vi "Global 6 Bool.vi"() -> ()   [LabVIEW 2022 SP3]
panel:
  out "Boolean":bool
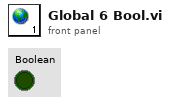
[diagram p1: front panel]
diagram:
